vi "Close_QuWire.vi"(8 "error in (no error)":errorcluster, 11 "QuWire in":refnum<class "QuWire.lvclass">) -> (0 "error out":errorcluster, 3 "QuWire out":refnum<class "QuWire.lvclass">)   [LabVIEW 2020, in "QuWire.lvclass"]
uses:
  QuWire.lvclass
  QuWire.lvclass/QuWire.ctl
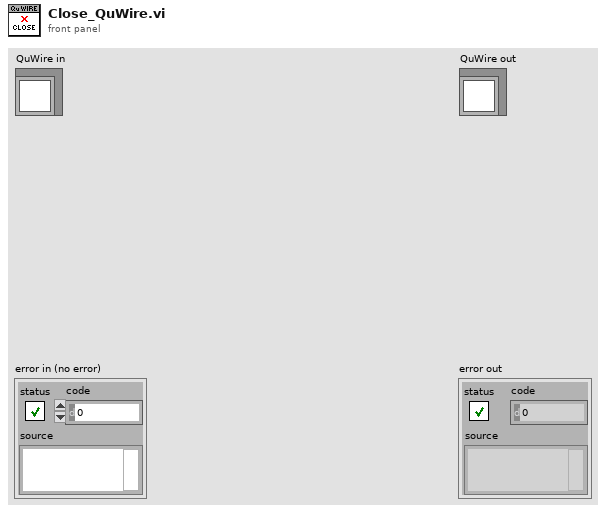
[diagram p1: front panel]
types:
  T1 = cluster{"List":refnum<queue>, "Update":refnum<notifier>}
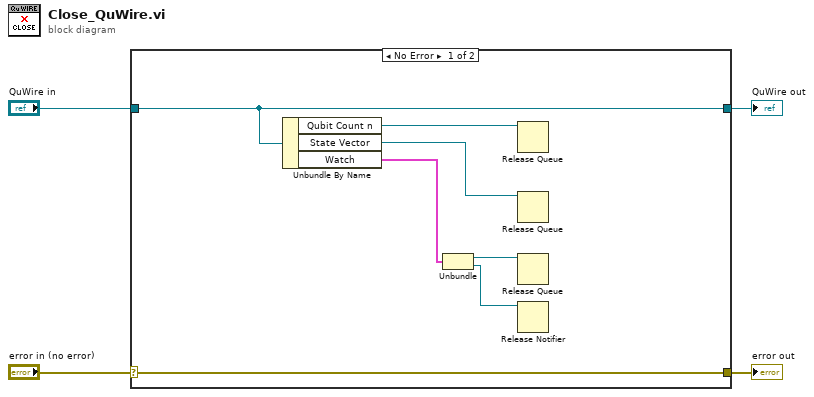
[diagram p0: block diagram]
diagram:
  n1 = case shown="No Error" "error in (no error)" {
    selector: "error in (no error)" -> [w11 w13]
    tunnel: [w11 w13] -> w3
    tunnel: [w8 w12] -> w1
    tunnel: "QuWire in" -> [w8 w12]
    frame No Error {
      n2 = Unbundle By Name(w8) -> ("Qubit Count n"=w10:refnum<queue>, "State Vector"=w9:refnum<queue>, "Watch"=w7:T1)
      n3 = Unbundle(w7) -> ("List"=w6:refnum<queue>, "Update"=w5:refnum<notifier>)
      n4 = Release Queue(queue=w10) -> ()  [unwired: 2 in, 3 out]
      n5 = Release Queue(queue=w9) -> ()  [unwired: 2 in, 3 out]
      n6 = Release Queue(queue=w6) -> ()  [unwired: 2 in, 3 out]
      n7 = Release Notifier(notifier=w5) -> ()  [unwired: 2 in, 3 out]
    }
    frame Error {
    }
  }
  "error out" <- w3
  "QuWire out" <- w1
